vi "aggiorna livello.vi"(10 "addendo":dbl, 11 "ARRAY SIM AI in":cluster{"Amplitude":dbl, "Precision %":dbl}[](array[cluster])) -> (3 "ARRAY SIM AI out":cluster{"Amplitude":dbl, "Precision %":dbl}[](array[cluster]))   [LabVIEW 2019]
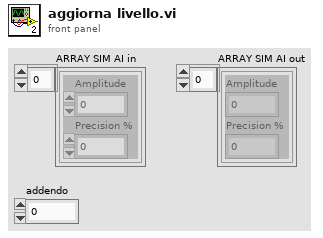
[diagram p1: front panel]
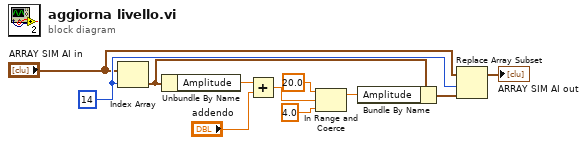
[diagram p0: block diagram]
diagram:
  w6 = 14 ("index")
  n1 = Index Array(array="ARRAY SIM AI in", index=w6) -> (element=w9:cluster{"Amplitude":dbl, "Precision %":dbl})
  n2 = Unbundle By Name(w9) -> ("Amplitude"=w7:dbl)
  n3 = Add(x=w7, y="addendo") -> (x+y=w4:dbl)
  n4 = In Range and Coerce(upper limit=20.0, x=w4, lower limit=4.0) -> (coerced(x)=w1:dbl)  [unwired: 1 out]
  n5 = Bundle By Name(cluster=w9, "Amplitude"=w1) -> (w10:cluster{"Amplitude":dbl, "Precision %":dbl})
  n6 = Replace Array Subset(array="ARRAY SIM AI in", new element=w10, index=w6) -> (→"ARRAY SIM AI out":cluster{"Amplitude":dbl, "Precision %":dbl}[])
